vi "Initialize.vi"(8 "error in":errorcluster, 9 "PPLs Folder Path":path, 10 "INI File Path":path, 11 "Device":string) -> (0 "error out":errorcluster, 3 "PLC out":refnum<class "PLC.lvclass">)   [LabVIEW 2018, in "PLC.lvlib" / "PLC.lvclass"]
uses:
  PLC.lvclass
  PLC.lvclass/PLC.ctl
  PPLs/Configuration/Configuration.lvlibp/Configuration.lvclass
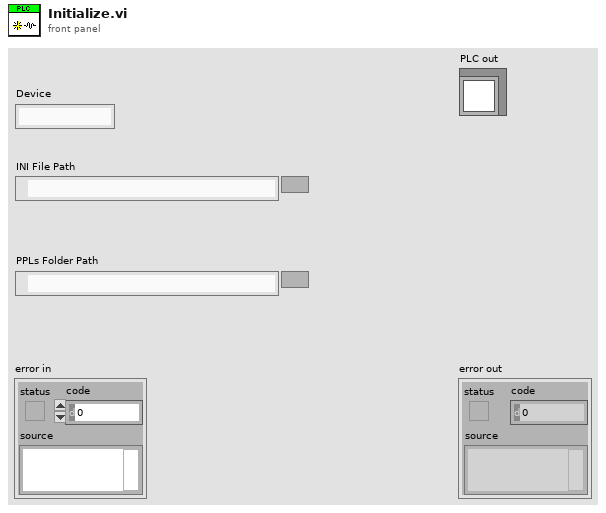
[diagram p1: front panel]
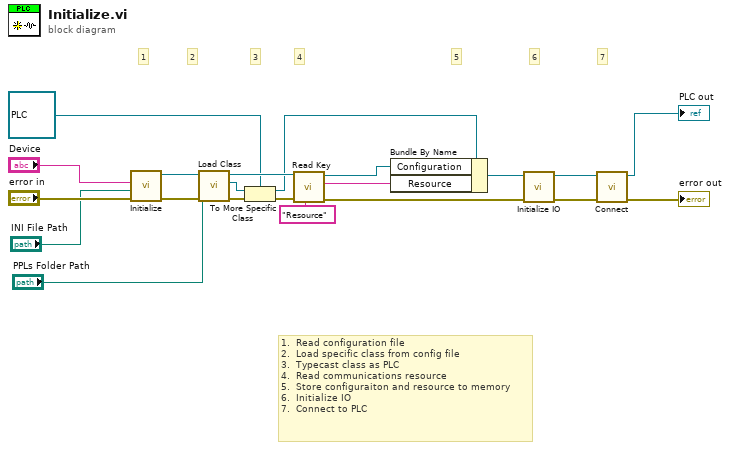
[diagram p0: block diagram]
diagram:
  # "1.  Read configuration file\n2.  Load specific class from config file\n3.  Typecast class as PLC\n4.  Read communications resource\n5.  Store configuraiton and resource to memory\n6.  Initialize IO\n7.  Connect to PLC"
  # "7"
  # "6"
  # "5"
  # "4"
  # "3"
  # "2"
  # "1"
  n1 = call "Initialize.vi"("error in"="error in", "INI File Path"="INI File Path", "Device"="Device") -> ("error out"=w18:errorcluster, "Configuration out"=w19:refnum<class "Configuration.lvclass">)  [unwired: 7 in]
  n2 = call "Load Class.vi"("error in"=w18, "PPLs Folder Path"="PPLs Folder Path", "Configuration in"=w19) -> ("error out"=w15:errorcluster, "Class out"=w14:refnum<class>, "Configuration out"=w17:refnum<class "Configuration.lvclass">)  [unwired: 6 in]
  n3 = To More Specific Class(target class=refnum<class "PLC.lvclass"> refnum ("PLC in"), reference=w14, error in=w15) -> (specific class reference=w7:refnum<class "PLC.lvclass">, error out=w12:errorcluster)
  n4 = call "Read Key.vi"("Key:"="Resource", "error in"=w12, "Configuration in"=w17) -> ("error out"=w3:errorcluster, "Value"=w4:string, "Configuration out"=w6:refnum<class "Configuration.lvclass">)  [unwired: 6 in]
  n5 = Bundle By Name(cluster=w7, "Configuration"=w6, "Resource"=w4) -> (w5:refnum<class "PLC.lvclass">)
  n6 = call "Initialize IO.vi"("error in"=w3, "PLC in"=w5) -> ("error out"=w8:errorcluster, "PLC out"=w9:refnum<class "PLC.lvclass">)  [unwired: 8 in]
  n7 = call-dynamic "Connect.vi"("error in (no error)"=w8, "PLC in"=w9) -> ("error out"=→"error out":errorcluster, "PLC out"=→"PLC out":refnum<class "PLC.lvclass">)  [unwired: 8 in]
